vi "11temp.vi"() -> ()   [LabVIEW 2013]
panel:
  out "Numeric":dbl
  out "Moderate Temperature":bool
  out "Low Temperature":bool
  out "High temperature":bool
  out "Meter":dbl(knob) scale=0.0..40.0
  in  "Temperature":dbl(slide) scale=0.0..40.0
  # "11.Temperature Monitoring"
  # "G SURESH\n23A91A0417\nECE-A"
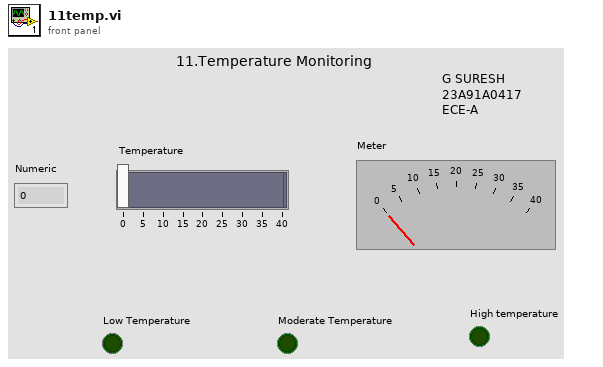
[diagram p1: front panel]
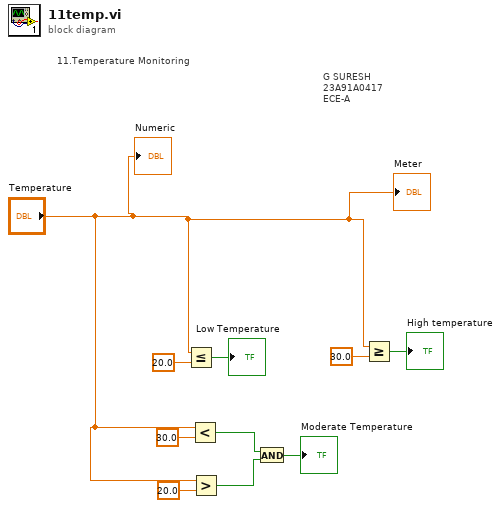
[diagram p0: block diagram]
diagram:
  # "G SURESH\n23A91A0417\nECE-A"
  # "11.Temperature Monitoring"
  n1 = Less Or Equal?(x="Temperature", y=20.0) -> (x <= y?=→"Low Temperature":bool)
  n2 = Less?(x="Temperature", y=30.0) -> (x < y?=w4:bool)
  n3 = Greater?(x="Temperature", y=20.0) -> (0:w3:bool)
  n4 = And(x=w4, y=w3) -> (x .and. y?=→"Moderate Temperature":bool)
  n5 = Greater Or Equal?(x="Temperature", y=30.0) -> (x >= y?=→"High temperature":bool)
  "Meter" <- "Temperature"
  "Numeric" <- "Temperature"
